vi "get_wavelengths_exp.vi"(8 "error in (no error)":errorcluster, 10 "Temp":bool, 11 "Experiment.lvclass in":refnum<class "Experiment.lvclass">) -> (0 "error out":errorcluster, 2 "wavelengths":dbl[](array[numeric]), 3 "Experiment.lvclass out":refnum<class "Experiment.lvclass">)   [LabVIEW 2020, in "Experiment.lvclass"]
uses:
  Experiment.lvclass
  Experiment.lvclass/Experiment.ctl
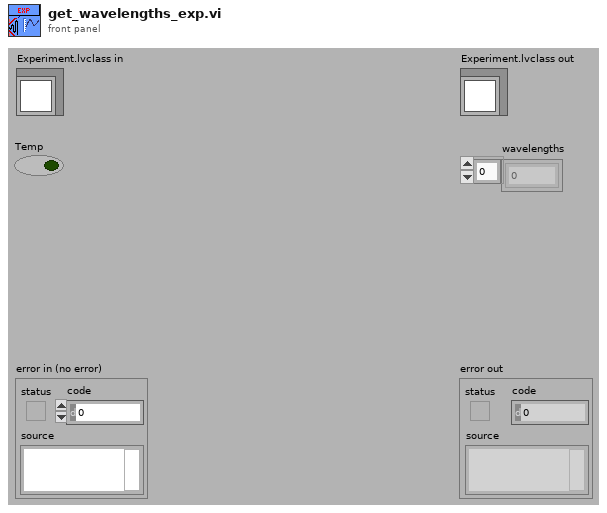
[diagram p1: front panel]
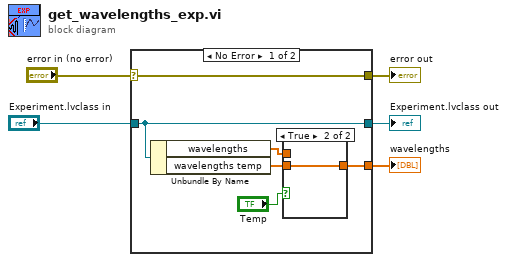
[diagram p0: block diagram]
diagram:
  n1 = case shown="No Error" "error in (no error)" {
    selector: "error in (no error)" -> [w11 w14]
    tunnel: [w11 w14] -> w4
    tunnel: [w10 w15] -> w2
    tunnel: "Experiment.lvclass in" -> [w10 w15]
    tunnel: [w8 _] -> w1
    frame No Error {
      n2 = Unbundle By Name(w10) -> ("wavelengths"=w9:dbl[], "wavelengths temp"=w6:dbl[])
      n3 = case shown="True" "Temp" {
        tunnel: [w12 w13] -> w8
        tunnel: w9 -> [w12 _]
        tunnel: w6 -> [_ w13]
        frame False {
        }
        frame True {
        }
      }
    }
    frame Error {
    }
  }
  "error out" <- w4
  "Experiment.lvclass out" <- w2
  "wavelengths" <- w1
